vi "Create All Message Queues.vi"(8 "error in (no error)":errorcluster caption="错误输入（无错误）") -> (0 "error out":errorcluster caption="错误输出", 3 "Message Queues out":T1 caption="消息队列输出")   [LabVIEW 2013, in "Message Queue.lvlib"]
doc: "本VI用于创建应用程序所需的所有消息队列。如应用程序需要两个以上消息队列，可右键单击上面的“消息队列”常量并选择“打开自定义类型”，将新的消息队列添加至该自定义类型，然后通过本VI进行初始化。"
uses:
  Message Queue.lvlib
  All Message Queues.ctl
  Message Cluster.ctl
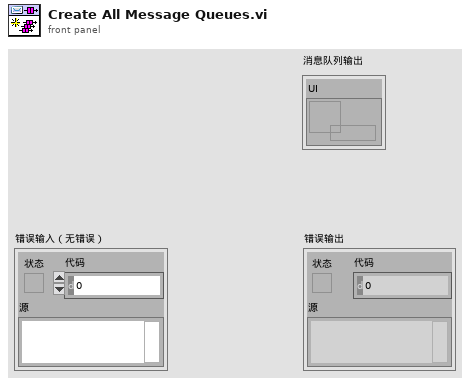
[diagram p1: front panel]
types:
  T1 = typedef "Message Queue.lvlib/All Message Queues.ctl" = cluster{"UI":refnum<queue>}
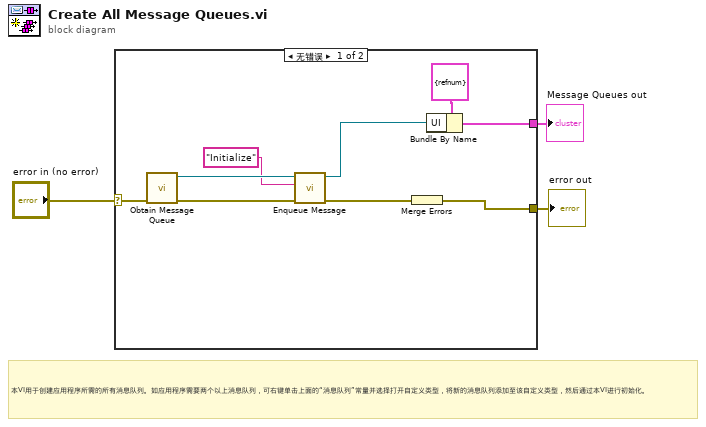
[diagram p0: block diagram]
diagram:
  # "本VI用于创建应用程序所需的所有消息队列。如应用程序需要两个以上消息队列，可右键单击上面的“消息队列”常量并选择打开自定义类型，将新的消息队列添加至该自定义类型，然后通过本VI进行初始化。"
  n1 = case shown="无错误" "error in (no error)" {
    selector: "error in (no error)" -> [w7 w13]
    tunnel: [w4 w13] -> w3
    tunnel: [w10 _] -> w2
    frame No Error {
      n2 = call "Obtain Message Queue.vi"("error in (no error)"=w7) -> ("error out"=w9:errorcluster, "Message Queue"=w8:refnum<queue>)  [unwired: 9 in]
      n3 = call "Enqueue Message.vi"("error in (no error)"=w9, "Message"="Initialize", "Message Queue"=w8) -> ("error out"=w12:errorcluster, "dup Message Queue"=w5:refnum<queue>)  [unwired: 7 in]
      n4 = Merge Errors(w12) -> (w4:errorcluster)
      n5 = Bundle By Name(cluster=T1 {"UI"=refnum} ("Message Queues"), "UI"=w5) -> (w10:T1)
    }
    frame Error {
    }
  }
  "Message Queues out" <- w2
  "error out" <- w3
